vi "Init Globals.vi"(8 "error in":errorcluster) -> (0 "error out":errorcluster, 3 "Events":T1)   [LabVIEW 2020, in "Netatmo-WeatherStation.lvlib"]
uses:
  Netatmo-WeatherStation.lvlib
  globals.vi
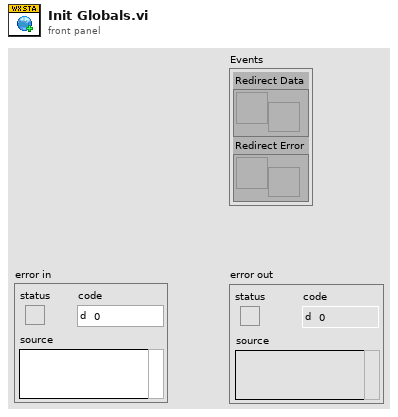
[diagram p1: front panel]
types:
  T1 = cluster{"Redirect Data":refnum<user-event>, "Redirect Error":refnum<user-event>}
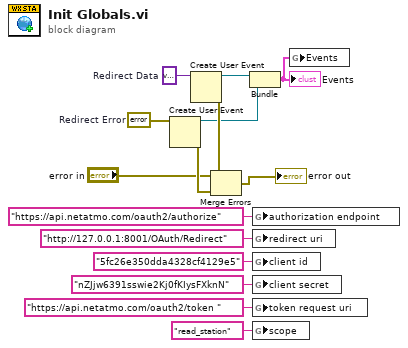
[diagram p0: block diagram]
diagram:
  w14 = errorcluster {"status"=FALSE, "code"=0, "source"=""}  # Redirect Error
  w15 = variant  # Redirect Data
  n1 = Create User Event(user event datatype=w14) -> (user event=w9:refnum<user-event>, error out=w13:errorcluster)  [unwired: 1 in]
  n2 = Create User Event(user event datatype=w15) -> (user event=w10:refnum<user-event>, error out=w11:errorcluster)  [unwired: 1 in]
  n3 = Merge Errors("error in", w11, w13) -> (→"error out":errorcluster)
  n4 = Bundle("Redirect Data"=w10, "Redirect Error"=w9) -> (w8:T1)  [unwired: 1 in]
  "Events" <- w8
  n5 = global write "globals.vi" "authorization endpoint"("https://api.netatmo.com/oauth2/authorize" ("authorization endpoint")) -> ()
  n6 = global write "globals.vi" "redirect uri"("http://127.0.0.1:8001/OAuth/Redirect" ("redirect uri")) -> ()
  n7 = global write "globals.vi" "client id"("5fc26e350dda4328cf4129e5" ("client id")) -> ()
  n8 = global write "globals.vi" "client secret"("nZJjw6391sswie2Kj0fKIysFXknN" ("client secret")) -> ()
  n9 = global write "globals.vi" "token request uri"("https://api.netatmo.com/oauth2/token " ("token request uri")) -> ()
  n10 = global write "globals.vi" "scope"("read_station" ("scope")) -> ()
  n11 = global write "globals.vi" "Events"(w8) -> ()
